vi "TCP Multiple Connections - Server.vi"() -> ()   [LabVIEW 2013]
doc: "该范例为支持客户端VI多个连接的TCP服务器VI。"
uses:
  controls/TCP Multiple Connections State.ctl
  controls/TCP Multiple Connections Data.ctl
panel:
  in  "停止":bool
  out "当前数据":dbl
  out "连接数":i32
  # "概述：演示使用TCP函数初始化可向多个客户端VI发送数据的TCP服务器。\n操作步骤：\n1. 运行VI。\n2. 打开TCP Multiple Connections - Client 1.vi并按照前面板上的说明操作。\n3. 打开TCP Multiple Connections - Client 2.vi并按照前面板上的说明操作。\n4. 单击停止可停止VI。"
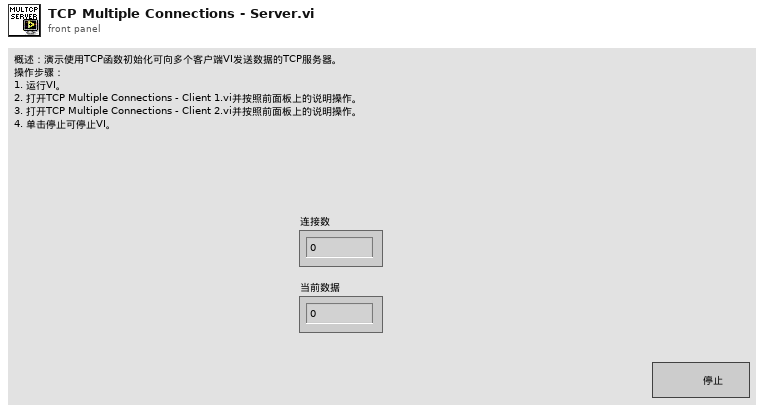
[diagram p1: front panel]
types:
  T1 = typedef "TCP Multiple Connections Data.ctl" = cluster{"客户端":refnum<k5>[], "侦听器":refnum<k5>}
  T2 = typedef "TCP Multiple Connections State.ctl" = enum16{"Initialize", "Status Check", "Send Data", "Stop"}
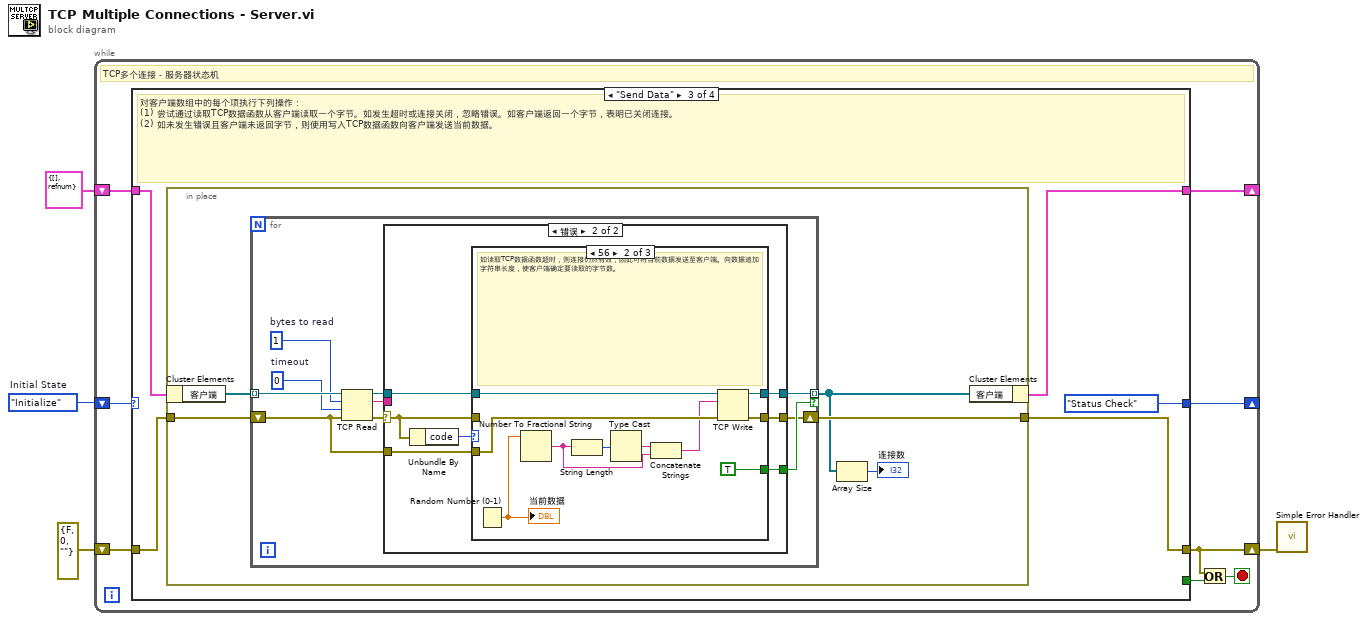
[diagram p0: block diagram]
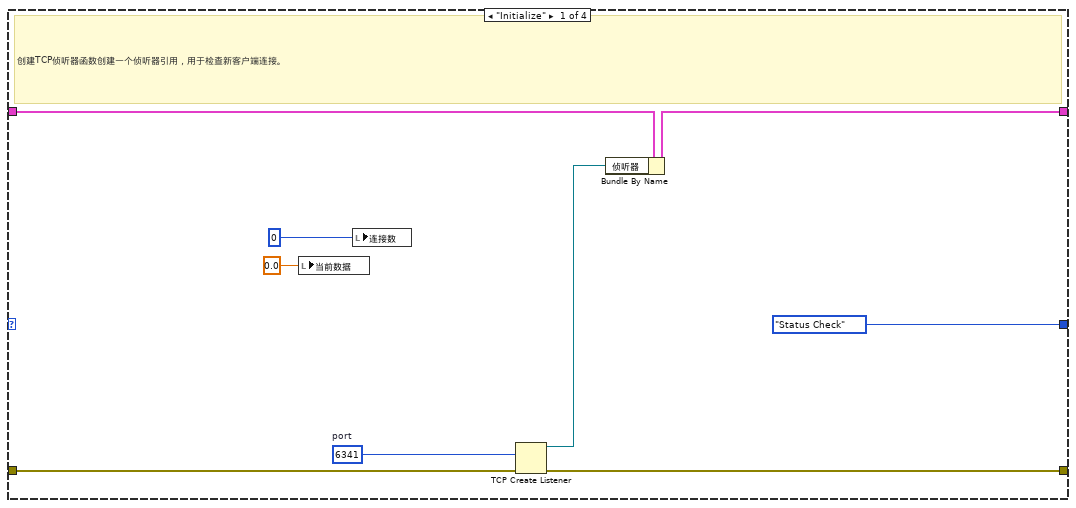
[diagram p2: hidden frame]
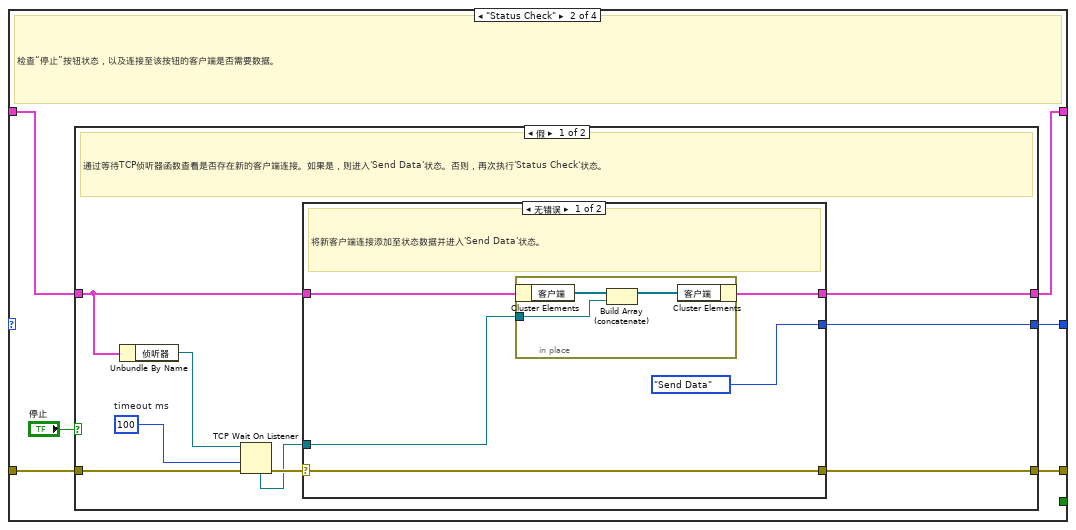
[diagram p3: hidden frame]
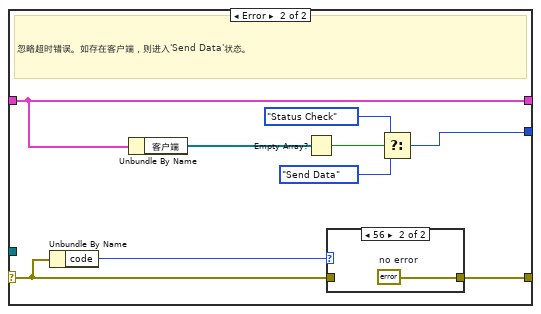
[diagram p4: hidden frame]
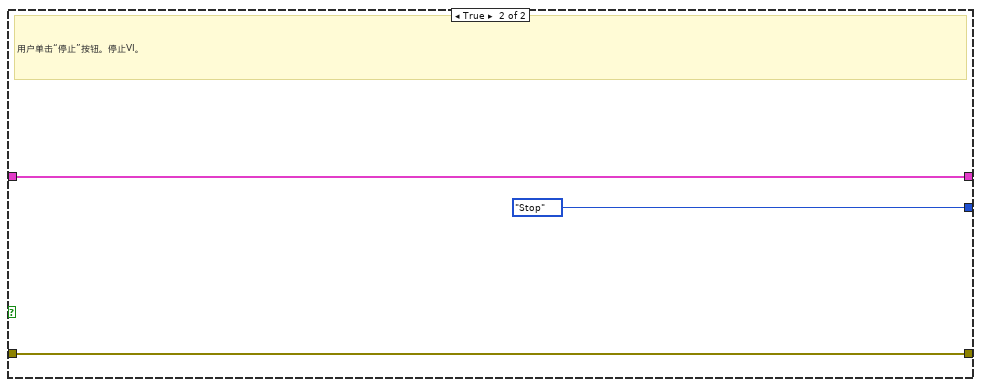
[diagram p6: hidden frame]
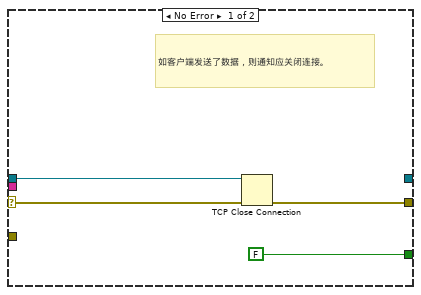
[diagram p7: hidden frame]
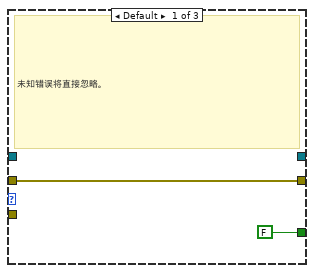
[diagram p8: hidden frame]
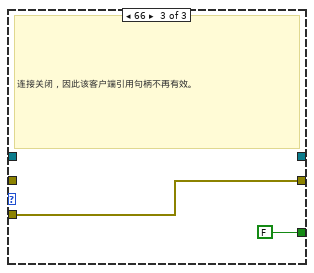
[diagram p9: hidden frame]
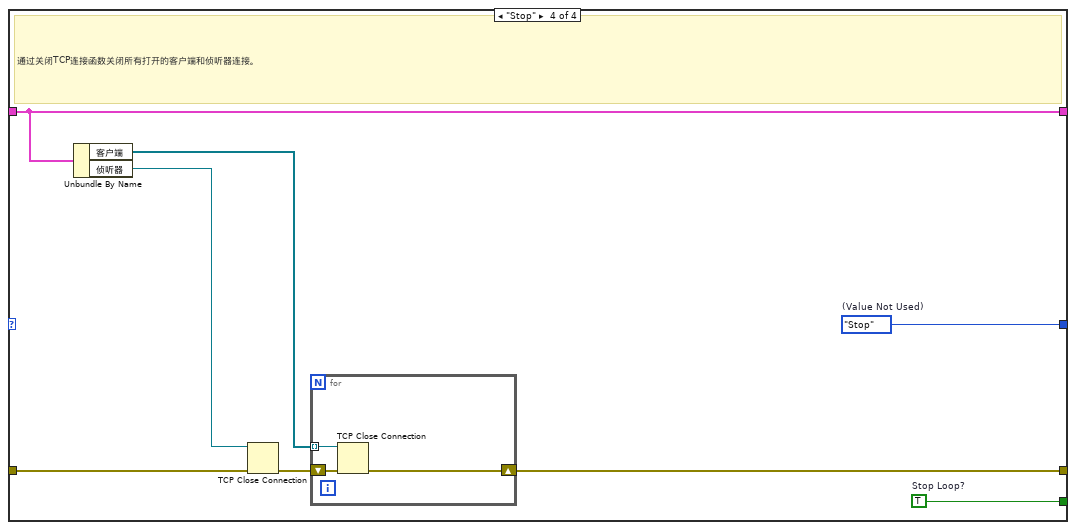
[diagram p10: hidden frame]
diagram:
  w4 = TCP_Multiple_Connections_State."Initialize"  # Initial State
  n1 = while {
    shift-right: [w11] -> _
    shift-left: w4 -> [w12]
    shift-right: [w9] -> _
    shift-left: T1 {"客户端"=[], "侦听器"=refnum} ("Data") -> [w10]
    shift-right: [w5] -> w1
    shift-left: errorcluster {"status"=FALSE, "code"=0, "source"=""} ("error constant") -> [w8]
    stop <- w6 stop-if-true
    # "TCP多个连接－服务器状态机"
    n2 = case shown="\"Send Data\"" w12 {
      tunnel: [TCP_Multiple_Connections_State."Status Check" ("States") w27 TCP_Multiple_Connections_State."Status Check" ("States") w104] -> w11
      tunnel: [_ _ _ w111] -> w7
      tunnel: w10 -> [w19 w23 w61 w110]
      tunnel: [w18 w22 w60 w110] -> w9
      tunnel: w8 -> [w21 w26 w63 w109]
      tunnel: [w20 w25 w62 w107] -> w5
      frame "Initialize" {
        w16 = u16 6341  # port
        # "创建TCP侦听器函数创建一个侦听器引用，用于检查新客户端连接。"
        n3 = local write "当前数据"(0.0 ("Current Data")) -> ()
        n4 = local write "连接数"(0 ("Number of Client Connections")) -> ()
        n5 = TCP Create Listener(8:w21, 10:w16) -> (0:w20:errorcluster, 3:w17:refnum<k5>)  [unwired: 4 out]
        n6 = Bundle By Name(cluster=w19, "侦听器"=w17) -> (w18:T1)
      }
      frame "Status Check" {
        # "检查“停止”按钮状态，以及连接至该按钮的客户端是否需要数据。"
        n7 = case shown="假" "停止" {
          tunnel: [w36 TCP_Multiple_Connections_State."Stop" ("States")] -> w27
          tunnel: w26 -> [w35 w58]
          tunnel: [w28 w58] -> w25
          tunnel: w23 -> [w31 w57]
          tunnel: [w30 w57] -> w22
          frame False {
            w34 = 100  # timeout ms
            # "通过等待TCP侦听器函数查看是否存在新的客户端连接。如果是，则进入'Send Data'状态。否则，再次执行'Status Check'状态。"
            n8 = Unbundle By Name(w31) -> ("侦听器"=w29:refnum<k5>)
            n9 = TCP Wait On Listener(8:w35, 9:w34, 11:w29) -> (0:w33:errorcluster, 4:w32:refnum<k5>)  [unwired: 4 out]
            n10 = case shown="无错误" w33 {
              selector: w33 -> [w39 w53]
              tunnel: [TCP_Multiple_Connections_State."Send Data" ("States") w47] -> w36
              tunnel: w32 -> [w40 _]
              tunnel: w31 -> [w41 w50]
              tunnel: [w38 w50] -> w30
              tunnel: [w39 w51] -> w28
              frame No Error {
                # "将新客户端连接添加至状态数据并进入'Send Data'状态。"
                n11 = in-place {
                  in-place-border: w40 -> [w42]
                  n12 = in-place-cluster #1(w41) -> ("客户端"=w44:refnum<k5>[])
                  n13 = Build Array (concatenate)(w44, w42) -> (w43:refnum<k5>[])
                  n14 = in-place-cluster #1("客户端"=w43) -> (w38:T1)
                }
              }
              frame Error {
                # "忽略超时错误。如存在客户端，则进入'Send Data'状态。"
                n15 = Unbundle By Name(w53) -> ("code"=w52:i32)
                n16 = Unbundle By Name(w50) -> ("客户端"=w49:refnum<k5>[])
                n17 = Empty Array?(array=w49) -> (empty?=w48:bool)
                n18 = case shown="56" w52 {
                  tunnel: w53 -> [w54 _]
                  tunnel: [w54 w55] -> w51
                  frame Default {
                  }
                  frame 56 {
                    w55 = errorcluster {"status"=FALSE, "code"=0, "source"=""}  # no error
                  }
                }
                n19 = Select(t=TCP_Multiple_Connections_State."Status Check" ("States"), s=w48, f=TCP_Multiple_Connections_State."Send Data" ("States")) -> (s? t:f=w47:T2)
              }
            }
          }
          frame True {
            # "用户单击“停止”按钮。停止VI。"
          }
        }
      }
      frame "Send Data" {
        # "对客户端数组中的每个项执行下列操作：\n(1) 尝试通过读取TCP数据函数从客户端读取一个字节。如发生超时或连接关闭，忽略错误。如客户端返回一个字节，表明已关闭连接。\n(2) 如未发生错误且客户端未返回字节，则使用写入TCP数据函数向客户端发送当前数据。"
        n20 = in-place {
          in-place-border: w63 -> [w68]
          in-place-border: [w67] -> w62
          n21 = in-place-cluster #2(w61) -> ("客户端"=w65:refnum<k5>[])
          n22 = for {
            tunnel: w65 -> [w78] mode=indexing
            shift-right: [w70] -> w67
            shift-left: w68 -> [w69]
            tunnel: [w72] -> w64 mode=indexing if=w71
            w75 = 0  # timeout
            w76 = 1  # bytes to read
            n23 = TCP Read(connection ID=w78, bytes to read=w76, error in (no error)=w69, 9:w75) -> (connection ID out=w77:refnum<k5>, data out=w73:string, error out=w74:errorcluster)  [unwired: 1 out]
            n24 = case shown="错误" w74 {
              selector: w74 -> [w81 w88]
              tunnel: w77 -> [w82 w85]
              tunnel: w73 -> [_ _]
              tunnel: [_ w83] -> w72
              tunnel: [FALSE w84] -> w71
              tunnel: [w79 w87] -> w70
              tunnel: w69 -> [_ w86]
              frame No Error {
                # "如客户端发送了数据，则通知应关闭连接。"
                # "如客户端发送了数据，则通知应关闭连接。"
                n25 = TCP Close Connection(connection ID=w82, error in (no error)=w81) -> (error out=w79:errorcluster)  [unwired: 2 out]
              }
              frame Error {
                # "忽略连接关闭和超时错误"
                n26 = Unbundle By Name(w88) -> ("code"=w89:i32)
                n27 = case shown="56" w89 {
                  tunnel: w88 -> [w91 _ _]
                  tunnel: [w91 w101 w103] -> w87
                  tunnel: w86 -> [_ w97 w103]
                  tunnel: w85 -> [_ w100 _]
                  tunnel: [FALSE TRUE FALSE] -> w84
                  tunnel: [_ w99 _] -> w83
                  frame Default {
                    # "未知错误将直接忽略。"
                  }
                  frame 56 {
                    # "如读取TCP数据函数超时，则连接仍然有效，因此可将当前数据发送至客户端。向数据追加字符串长度，使客户端确定要读取的字节数。"
                    n28 = Random Number (0-1)() -> (number: 0 to 1=w96:dbl)
                    "当前数据" <- w96
                    n29 = Number To Fractional String(number=w96) -> (F-format string=w93:string)  [unwired: 3 in]
                    n30 = String Length(string=w93) -> (length=w94:i32)
                    n31 = Type Cast(x=w94) -> (*(type *) &x=w95:string)  [unwired: 1 in]
                    n32 = Concatenate Strings(w95, w93) -> (w92:string)
                    n33 = TCP Write(connection ID=w100, data in=w92, error in (no error)=w97) -> (connection ID out=w99:refnum<k5>, error out=w101:errorcluster)  [unwired: 2 out]
                  }
                  frame 66 {
                    # "连接关闭，因此该客户端引用句柄不再有效。"
                  }
                }
              }
            }
          }
          n34 = Array Size(array=w64) -> (size(s)=→"连接数":i32)
          n35 = in-place-cluster #2("客户端"=w64) -> (w60:T1)
        }
      }
      frame "Stop" {
        w104 = TCP_Multiple_Connections_State."Stop"  # (Value Not Used)
        w111 = TRUE  # Stop Loop?
        # "通过关闭TCP连接函数关闭所有打开的客户端和侦听器连接。"
        n36 = Unbundle By Name(w110) -> ("客户端"=w108:refnum<k5>[], "侦听器"=w105:refnum<k5>)
        n37 = TCP Close Connection(connection ID=w105, error in (no error)=w109) -> (error out=w106:errorcluster)  [unwired: 1 in, 1 out]
        n38 = for {
          shift-right: [w113] -> w107
          shift-left: w106 -> [w114]
          tunnel: w108 -> [w112] mode=indexing
          n39 = TCP Close Connection(connection ID=w112, error in (no error)=w114) -> (error out=w113:errorcluster)  [unwired: 1 in, 1 out]
        }
      }
    }
    n40 = Or(x=w5, y=w7) -> (x .or. y?=w6:bool)
  }
  n41 = call <vilib>:"Simple Error Handler.vi"("error in (no error)"=w1) -> ()  [unwired: 4 in, 5 out]
